vi "003LockerComboAnsA.vi"() -> ()   [LabVIEW 2010]
panel:
  out "Can Open?":bool
  in  "#4":i32
  in  "#3":i32
  in  "#2":i32
  in  "#1":i32
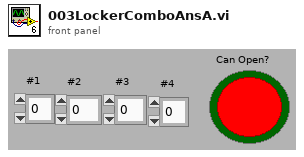
[diagram p1: front panel]
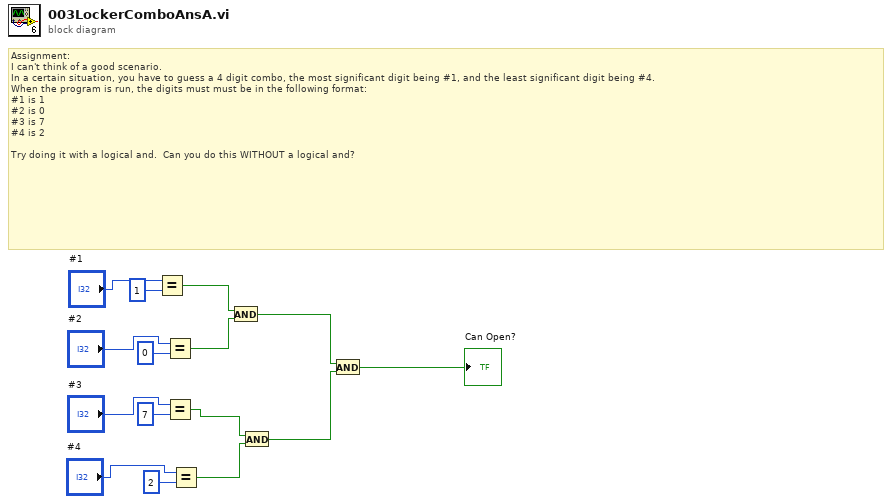
[diagram p0: block diagram]
diagram:
  # "Assignment:\nI can't think of a good scenario.\nIn a certain situation, you have to guess a 4 digit combo, the most significant digit being #1, and the least significant digit being #4.\nWhen the program is run, the digits must must be in the following format:\n#1 is 1\n#2 is 0\n#3 is 7\n#4 is 2\n\nTry doing it with a logical and.  Can you do this WITHOUT a logical and?"
  n1 = Equal?(x="#1", y=1) -> (x = y?=w7:bool)
  n2 = Equal?(x="#2", y=0) -> (x = y?=w6:bool)
  n3 = Equal?(x="#3", y=7) -> (x = y?=w5:bool)
  n4 = Equal?(x="#4", y=2) -> (x = y?=w4:bool)
  n5 = And(x=w7, y=w6) -> (x .and. y?=w2:bool)
  n6 = And(x=w5, y=w4) -> (x .and. y?=w3:bool)
  n7 = And(x=w2, y=w3) -> (x .and. y?=→"Can Open?":bool)
